vi "Reset.vi"(8 "error in":errorcluster, 11 "lia rt in":refnum<class "Lock-In Amplifier Example RT.lvclass">) -> (0 "error out":errorcluster, 3 "lia rt out":refnum<class "Lock-In Amplifier Example RT.lvclass">)   [LabVIEW 2017, in "Lock-In Amplifier Example RT.lvclass"]
uses:
  Lock-In Amplifier Example RT.lvclass
  Properties/FpgaSession_GET.vi
  interface/Interface FPGA/LIA Host Interface FPGA.lvclass
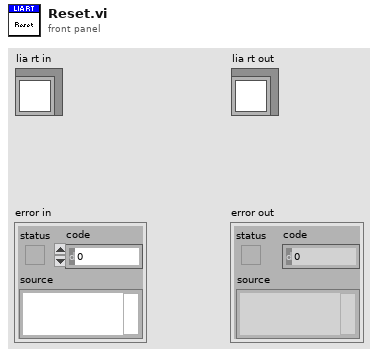
[diagram p1: front panel]
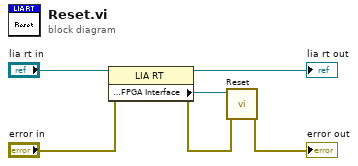
[diagram p0: block diagram]
diagram:
  n1 = property class="LIA RT"(reference="lia rt in", error in="error in") -> (reference out=→"lia rt out":refnum<class "Lock-In Amplifier Example RT.lvclass">, error out=w2:errorcluster, "Properties:FPGA Interface"=w3:refnum<class "LIA Host Interface FPGA.lvclass">)
  n2 = call-dynamic "Reset.vi"("error in"=w2, "host in"=w3) -> ("error out"=→"error out":errorcluster)  [unwired: 8 in, 1 out]
